vi "二值化(子VI).vi"(11 "引用句柄输入":T1) -> (2 "Image Dst Out":T1, 3 "引用句柄输出":T1(plugin-control))   [LabVIEW 2012]
uses:
  <vilib>/vision/Image Controls.llb/IMAQ Image.ctl
  <vilib>/vision/NI_Vision_Development_Module.lvlib
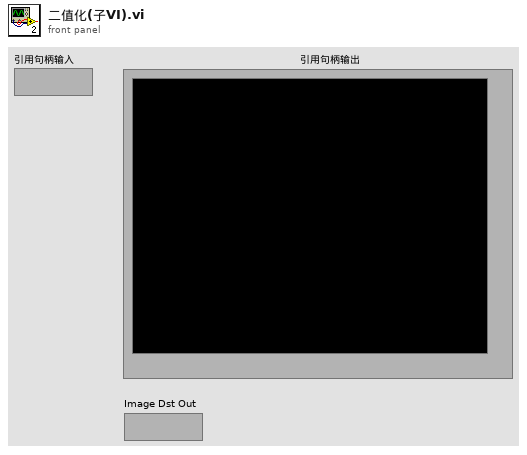
[diagram p1: front panel]
types:
  T1 = typedef "IMAQ Image.ctl" = refnum<image>
  T2 = typedef "Image Type" = u32
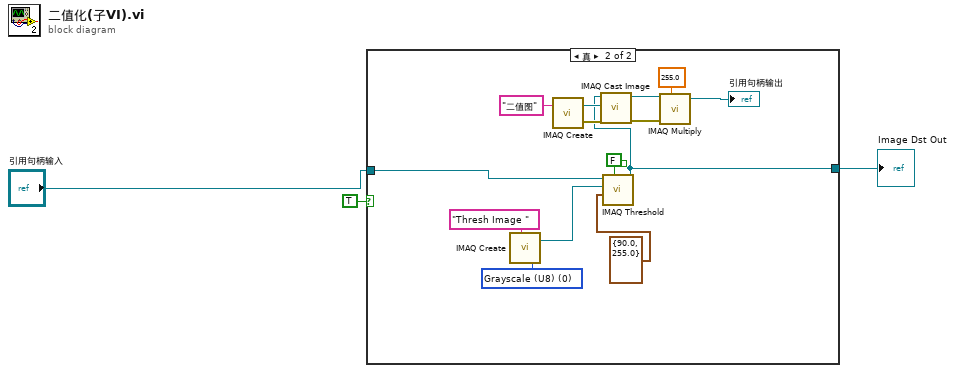
[diagram p0: block diagram]
diagram:
  n1 = case shown="真" TRUE {
    tunnel: "引用句柄输入" -> [w4 w7]
    tunnel: [w4 w6] -> w2
    frame False {
    }
    frame True {
      w10 = T2 0 items=["Grayscale (U8)", "Grayscale (I16)", "Grayscale (SGL)", "Complex (CSG)", "RGB (U32)", "HSL (U32)", "RGB (U64)", "Grayscale (U16)"] ("Image Type")
      n2 = call "IMAQ Create"("Image Name"="Thresh Image ", "Image Type"=w10) -> ("New Image"=w17:T1)  [unwired: 3 in, 1 out]
      n3 = call "IMAQ Create"("Image Name"="二值图") -> ("New Image"=w13:T1, "error out"=w12:errorcluster)  [unwired: 4 in]
      n4 = call "IMAQ Threshold"("Keep/Replace Value (Replace)"=FALSE, "Range"=cluster{"Lower value":sgl, "Upper value":sgl} {"Lower value"=90.0, "Upper value"=255.0} ("Range 2"), "Image Dst"=w17, "Image Src"=w7) -> ("Image Dst Out"=w6:T1)  [unwired: 6 in, 1 out]
      n5 = call "IMAQ Cast Image"("error in (no error)"=w12, "Image Dst"=w13, "Image Src"=w6) -> ("error out"=w15:errorcluster, "Image Dst Out"=w14:T1)  [unwired: 7 in]
      n6 = call "IMAQ Multiply"("Image Src A"=w14, "Constant"=sgl 255.0, "error in (no error)"=w15) -> ("Image Dst Out"=→"引用句柄输出":T1)  [unwired: 4 in, 1 out]
    }
  }
  "Image Dst Out" <- w2
